vi "Find Target Actor.vi"(5 "Target":refnum<vi>, 7 "App Inst":refnum<vi>, 8 "error in (no error)":errorcluster, 11 "Message Path":path) -> (0 "error out":errorcluster, 3 "Targeted Actor":path)   [LabVIEW 2020, in "Message Rescripter.lvlib"]
uses:
  Message Rescripter.lvlib
  <vilib>/Utility/traverseref.llb/TRef TravTarget.ctl
  <vilib>/ErrorRing/Error Ring.xnode
  <vilib>/Utility/traverseref.llb/VI Scripting - Traverse.lvlib
  <vilib>/Utility/Data Type/NI_Data Type.lvlib
  MessageMakerProvider/AFPP Shared/AFPP Shared.lvlib
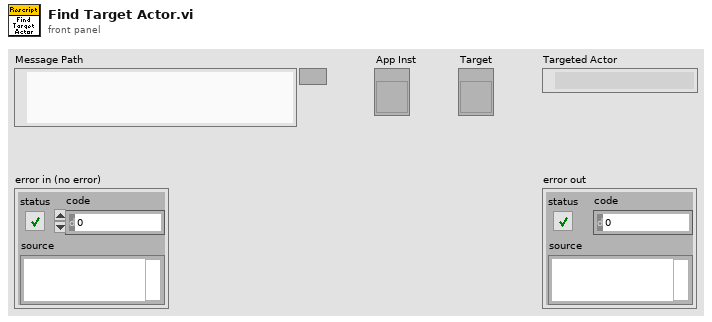
[diagram p1: front panel]
types:
  T1 = typedef "TRef TravTarget.ctl" = enum16{"FP", "BD", "Other"}
  T2 = typedef "NI_FileType.lvlib/LVFileType.ctl" = enum32{"Invalid file", "Unknown type", "Instrument", "Control", "Polymorphic VI", "Project", "Library", "LVClass", "XControl", "XNode", "Shared library", ".NET assembly", "ActiveX interface", "CIN", "Run-time menu", "Palette menu", "Help file", "LLB", "XNode Edit Dependency", "Class Private Data Control", "Statechart", "MathScript .m file", "Ladder Diagram", "LVLibp", "XNode Build Dependency"}
  T3 = cluster{"path":path, "delimited name":string, "type":T2}[]
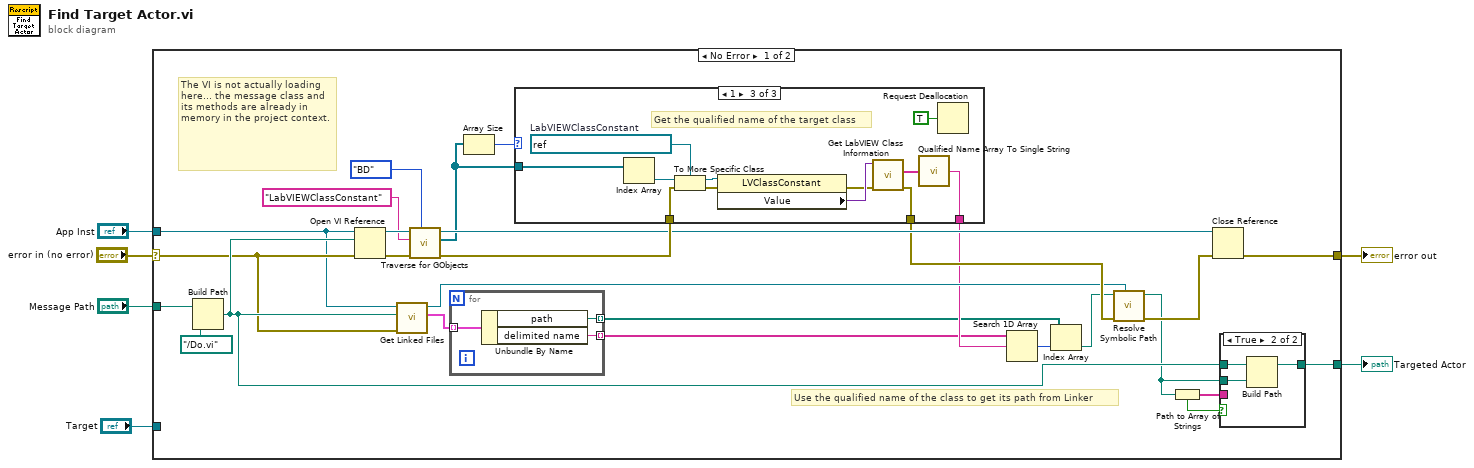
[diagram p0: block diagram]
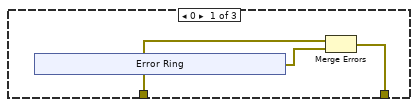
[diagram p2: hidden frame]
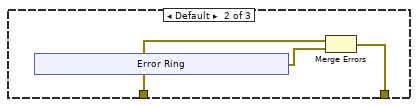
[diagram p3: hidden frame]
diagram:
  n1 = case shown="No Error" "error in (no error)" {
    selector: "error in (no error)" -> [w30 w61]
    tunnel: "Message Path" -> [w33 _]
    tunnel: [w10 _] -> w5
    tunnel: "App Inst" -> [w14 _]
    tunnel: [w29 w61] -> w3
    tunnel: "Target" -> [_ _]
    frame No Error {
      # "Use the qualified name of the class to get its path from Linker"
      # "The VI is not actually loading here... the message class and its methods are already in memory in the project context."
      n2 = Build Path(base path=w33, name or relative path=path "../Do.vi") -> (appended path=w31:path)
      n3 = Open VI Reference(application reference (local)=w14, vi path=w31, error in (no error)=w30) -> (vi reference=w28:refnum<vi>, error out=w27:errorcluster)  [unwired: 3 in]
      n4 = call "Get Linked Files.vi"("error in (no error)"=w30, "File path"=w31, "Application in"=w14) -> ("Linked Files"=w9:T3, "Application out"=w20:refnum<vi>)  [unwired: 7 in]
      n5 = call <vilib>:"Traverse for GObjects.vi"("Traverse Target"=TRef_TravTarget."BD", "error in (no error)"=w27, "Class Name"="LabVIEWClassConstant", "VI Refnum"=w28) -> ("error out"=w24:errorcluster, "References"=w13:refnum<vi>[], "dup VI Refnum"=w23:refnum<vi>)  [unwired: 4 in, 1 out]
      n6 = for {
        tunnel: w9 -> [w36] mode=indexing
        tunnel: [w35] -> w8 mode=indexing
        tunnel: [w34] -> w7 mode=indexing
        n7 = Unbundle By Name(w36) -> ("path"=w34:path, "delimited name"=w35:string)
      }
      n8 = Array Size(array=w13) -> (size(s)=w12:i32)
      n9 = case shown="1" w12 {
        tunnel: w24 -> [w39 w43 w54]
        tunnel: [w38 w42 w49] -> w21
        tunnel: [_ _ w47] -> w11
        tunnel: w13 -> [_ _ w45]
        frame 0 {
          n10 = xnode "Error Ring"() -> ("error out"=w37:errorcluster)
          n11 = Merge Errors(w39, w37) -> (w38:errorcluster)
        }
        frame Default {
          n12 = xnode "Error Ring"() -> ("error out"=w41:errorcluster)
          n13 = Merge Errors(w43, w41) -> (w42:errorcluster)
        }
        frame 1 {
          w56 = refnum<vi> refnum  # LabVIEWClassConstant
          # "Get the qualified name of the target class"
          n14 = Index Array(array=w45) -> (element=w52:refnum<vi>)  [unwired: 1 in]
          n15 = To More Specific Class(target class=w56, reference=w52, error in=w54) -> (specific class reference=w55:refnum<vi>, error out=w53:errorcluster)
          n16 = property class="LVClassConstant"(reference=w55, error in=w53) -> (error out=w50:errorcluster, "Value"=w51:variant)  [unwired: 1 out]
          n17 = call <vilib>:"Get LabVIEW Class Information.vi"("error in (no error)"=w50, "variant"=w51) -> ("error out"=w49:errorcluster, "qualified LabVIEW class name"=w48:string[])  [unwired: 7 in, 1 out]
          n18 = call <vilib>:"Qualified Name Array To Single String.vi"("Fully Qualified Array"=w48) -> ("Fully Qualified String"=w47:string)
          n19 = Request Deallocation(TRUE ("flag")) -> ()
        }
      }
      n20 = Search 1D Array(1D array=w8, element=w11) -> (index of element=w22:i32)  [unwired: 1 in]
      n21 = Index Array(array=w7, index=w22) -> (element=w19:path)
      n22 = call "Resolve Symbolic Path.vi"("App Inst"=w20, "error in (no error)"=w21, "Path"=w19) -> ("error out"=w18:errorcluster, "Resolved Path"=w15:path)  [unwired: 7 in]
      n23 = Path to Array of Strings(0:w15) -> (1:w16:bool, 2:w17:string[])
      n24 = Close Reference(reference=w23, error in (no error)=w18) -> (error out=w29:errorcluster)
      n25 = case shown="True" w16 {
        tunnel: w15 -> [w57 w58]
        tunnel: w17 -> [_ _]
        tunnel: w31 -> [_ w60]
        tunnel: [w57 w59] -> w10
        frame False {
        }
        frame True {
          n26 = Build Path(base path=w60, name or relative path=w58) -> (appended path=w59:path)
        }
      }
    }
    frame Error {
    }
  }
  "Targeted Actor" <- w5
  "error out" <- w3
